vi "Timetomatch.vi"() -> ()   [LabVIEW 2020]
doc: "This VI is the solution to an exercise in the LabVIEW Basics I course.\n\nIt is used to demonstrate passing data out of a while loop through a tunnel. This VI generates random numbers until the generated number matches a specified value. The loop count terminal keeps track of the number of iterations before a match occurs."
panel:
  out "Time to match":dbl format="%#_3g"
  in  "Number to Match":i32=50 min=0 max=10000 step=1
  out "# of iterations":i32
  out "Current Number":i32
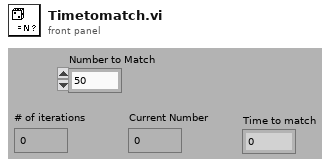
[diagram p1: front panel]
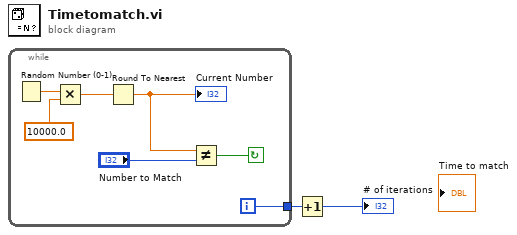
[diagram p0: block diagram]
diagram:
  n1 = while {
    tunnel: [w4] -> w2
    i -> [w4]
    stop <- w5 continue-if-true
    n2 = Random Number (0-1)() -> (number: 0 to 1=w6:dbl)
    n3 = Multiply(x=w6, y=10000.0) -> (x*y=w8:dbl)
    n4 = Round To Nearest(number=w8) -> (nearest integer value=w9:dbl)
    "Current Number" <- w9
    n5 = Not Equal?(x=w9, y="Number to Match") -> (x != y?=w5:bool)
  }
  n6 = Increment(x=w2) -> (x+1=→"# of iterations":i32)
